vi "Write HaltRole 5.vi"(8 "error in (no error)":errorcluster, 10 "HaltRole":refnum<class "HaltRole.lvclass">, 11 "HaltPlay in":refnum<class "HaltPlay.lvclass">) -> (0 "error out":errorcluster, 3 "HaltPlay out":refnum<class "HaltPlay.lvclass">)   [LabVIEW 2018, in "HaltPlay.lvclass"]
uses:
  HaltPlay.lvclass
  HaltRole_class/HaltRole.lvclass
  HaltPlay.lvclass/HaltPlay.ctl
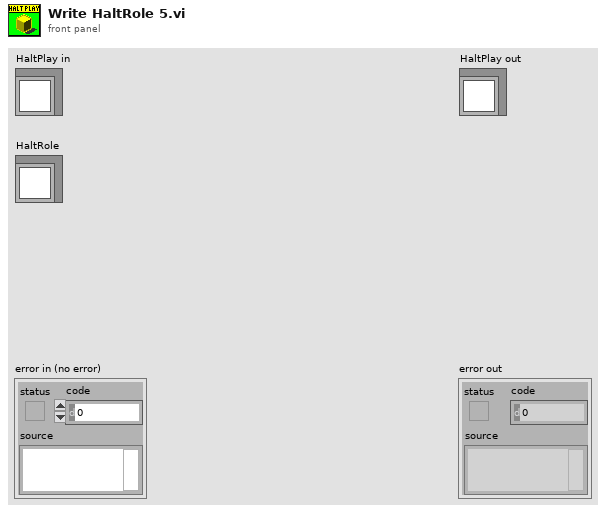
[diagram p1: front panel]
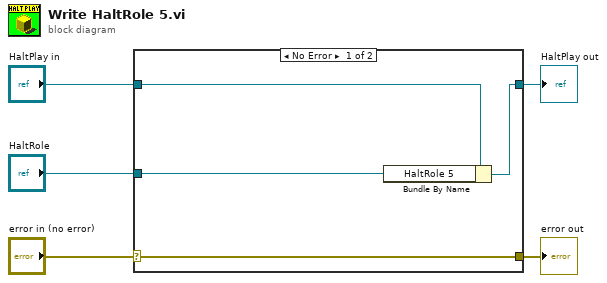
[diagram p0: block diagram]
diagram:
  n1 = case shown="No Error" "error in (no error)" {
    selector: "error in (no error)" -> [w9 w10]
    tunnel: [w9 w10] -> w4
    tunnel: [w7 w11] -> w2
    tunnel: "HaltPlay in" -> [w8 w11]
    tunnel: "HaltRole" -> [w6 _]
    frame No Error {
      n2 = Bundle By Name(cluster=w8, "HaltRole 5"=w6) -> (w7:refnum<class "HaltPlay.lvclass">)
    }
    frame Error {
    }
  }
  "error out" <- w4
  "HaltPlay out" <- w2
